vi "Range Plots.vi"(11 "Ranges":T1) -> (3 "Range Plots":cluster{sgl[], sgl[]}[](graph))   [LabVIEW 2020, in "FormulaG-Common.lvlib"]
uses:
  FormulaG-Common.lvlib
  Ranges.ctl
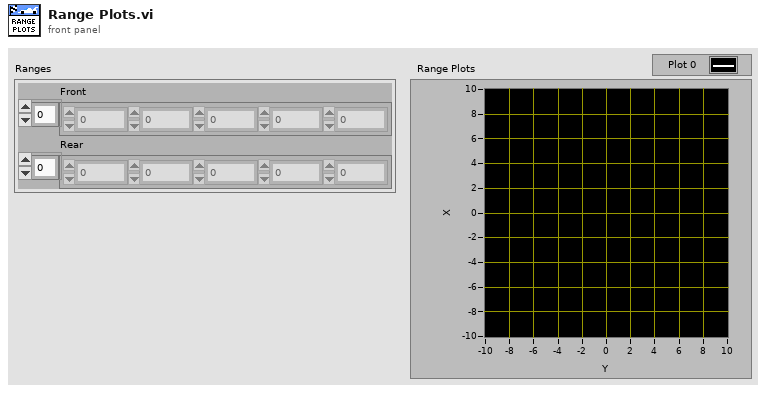
[diagram p1: front panel]
types:
  T1 = typedef "FormulaG-Common.lvlib/Ranges.ctl" = cluster{"Front":sgl[], "Rear":sgl[]}
  T2 = typedef "FormulaG-Common.lvlib/Point.ctl" = cluster{"X":sgl, "Y":sgl, "Frame":T3}
  T3 = typedef "FormulaG-Common.lvlib/Coordinate Frame.ctl" = enum16{"Global", "Local"}
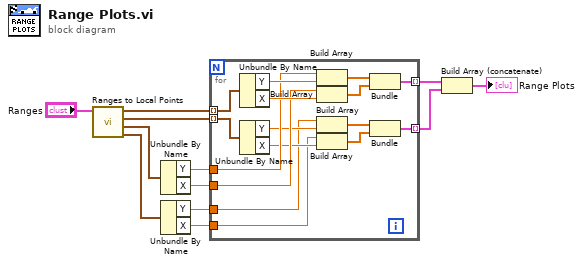
[diagram p0: block diagram]
diagram:
  n1 = call "Ranges to Local Points.vi"("Ranges"="Ranges") -> ("Rear Range Offset"=w8:T2, "Front Range Offset"=w9:T2, "Rear Points"=w10:T2[], "Front Points"=w11:T2[])  [unwired: 7 in]
  n2 = Unbundle By Name(w9) -> ("Y"=w6:sgl, "X"=w4:sgl)
  n3 = Unbundle By Name(w8) -> ("Y"=w7:sgl, "X"=w5:sgl)
  n4 = for {
    tunnel: w11 -> [w28] mode=indexing
    tunnel: w10 -> [w27] mode=indexing
    tunnel: w6 -> [w24]
    tunnel: w7 -> [w20]
    tunnel: w5 -> [w19]
    tunnel: w4 -> [w23]
    tunnel: [w14] -> w3 mode=indexing
    tunnel: [w13] -> w2 mode=indexing
    n5 = Unbundle By Name(w28) -> ("Y"=w26:sgl, "X"=w25:sgl)
    n6 = Unbundle By Name(w27) -> ("Y"=w22:sgl, "X"=w21:sgl)
    n7 = Build Array(w24, w26) -> (w18:sgl[])
    n8 = Build Array(w23, w25) -> (w17:sgl[])
    n9 = Build Array(w20, w22) -> (w16:sgl[])
    n10 = Build Array(w19, w21) -> (w15:sgl[])
    n11 = Bundle(w18, w17) -> (w14:cluster{sgl[], sgl[]})  [unwired: 1 in]
    n12 = Bundle(w16, w15) -> (w13:cluster{sgl[], sgl[]})  [unwired: 1 in]
  }
  n13 = Build Array (concatenate)(w3, w2) -> (→"Range Plots":cluster{sgl[], sgl[]}[])
